vi "PJ1_GG - Sigwork.vi"() -> ()   [LabVIEW 2024]
uses:
  Control 1.ctl
  <vilib>/Instr/_visa.llb/VISA Configure Serial Port (Instr).vi
  <vilib>/express/express analysis/Spectral/Block/exnSpectralBlock spectral measurements PSD poly.vi
  <vilib>/express/express analysis/Spectral/Block/exnSpectralBlock spectral measurements PSD DDT.vi
  <vilib>/express/express analysis/Spectral/XNode/ExpressSpectralMeasurementsBlockNode.xnode
panel:
  out "Array":dbl[](array[numeric])
  out "appended array 2":dbl[](array[numeric])
  out "data out":string
  in  "Sample":i32
  in  "Rate":dbl
  in  "Upper Cut-Off":dbl=40.0
  out "PSD":dynamicdata(graph)
  out "PSD MAX":dbl
  out "Index ที่มากที่สุด":i32
  out "max value":dbl
  out "B 18+1":dbl
  out "N 18+1":dbl
  in  "Aj 18+1":dbl
  out "B 18+1":dbl
  out "PSD 18+1":dbl
  out "B 18":dbl
  out "N 18":dbl
  in  "Aj 18":dbl
  out "B 18":dbl
  out "PSD 18":dbl
  out "B 18-1":dbl
  out "N 18-1":dbl
  in  "Aj 18-1":dbl
  out "B 18-1":dbl
  out "PSD 18-1":dbl
  out "9 Hz":dbl[](array[numeric])
  out "Max Index 9":i32
  out "PSD max 9":dbl
  out "PSD 9-1":dbl
  out "B 9-1":dbl
  in  "Aj 9-1":dbl
  out "N 9-1":dbl
  out "B 9-1":dbl
  out "PSD 9":dbl
  out "B 9":dbl
  in  "Aj 9":dbl
  out "N 9":dbl
  out "B 9":dbl
  out "PSD 9+1":dbl
  out "B 9+1":dbl
  in  "Aj 9+1":dbl
  out "N 9+1":dbl
  out "B 9+1":dbl
  out "8 Hz":dbl[](array[numeric])
  out "Max Index 8":i32
  out "PSD max 8":dbl
  out "B 16+1":dbl
  out "N 16+1":dbl
  in  "Aj  16+1":dbl
  out "B 16+1":dbl
  out "PSD  16+1":dbl
  out "B 16":dbl
  out "N  16":dbl
  in  "Aj  16":dbl
  out "B 16":dbl
  out "PSD  16":dbl
  out "B 16-1":dbl
  out "N  16-1":dbl
  in  "Aj   16-1":dbl
  out "B   16-1":dbl
  out "PSD 16-1":dbl
  out "B 8+1":dbl
  out "N 8+1":dbl
  in  "Aj  8+1":dbl
  out "B  8+1":dbl
  out "PSD 8+1":dbl
  out "B 8":dbl
  out "N  8":dbl
  in  "Aj  8":dbl
  out "B  8":dbl
  out "PSD 8":dbl
  out "B 8-1":dbl
  out "N  8-1":dbl
  in  "Aj  8-1":dbl
  out "B  8-1":dbl
  out "PSD 8-1":dbl
  out "PSD 14+1":dbl
  out "B 14+1":dbl
  in  "Aj 14+1":dbl
  out "N 14+1":dbl
  out "B 14+1":dbl
  out "PSD 14":dbl
  out "B 14":dbl
  in  "Aj 14":dbl
  out "N 14":dbl
  out "B 14":dbl
  out "PSD 14-1":dbl
  out "B 14-1":dbl
  in  "Aj 14-1":dbl
  out "N 14-1":dbl
  out "B 14-1":dbl
  out "PSD7+1":dbl
  out "B7+1":dbl
  in  "Aj7+1":dbl
  out "N7+1":dbl
  out "B7+1":dbl
  out "PSD 7":dbl
  out "B 7":dbl
  in  "Aj 7":dbl
  out "N7":dbl
  out "B7":dbl
  out "7 Hz":dbl[](array[numeric])
  out "Max Index 7":i32
  out "PSD max 7":dbl
  out "PSD 7-1":dbl
  out "B 7-1":dbl
  in  "Aj 7-1":dbl
  out "N7-1":dbl
  out "B7-1":dbl
  out "B12-1":dbl
  out "N12-1":dbl
  in  "Aj 12-1":dbl
  out "B 12-1":dbl
  out "PSD 12-1":dbl
  out "B12":dbl
  out "N12":dbl
  in  "Aj 12":dbl
  out "B12":dbl
  out "PSD 12":dbl
  out "B12+1":dbl
  out "N12+1":dbl
  in  "Aj 12+1":dbl
  out "B 12+1":dbl
  out "PSD 12+1":dbl
  out "B6+1":dbl
  out "N6+1":dbl
  in  "Aj 6+1":dbl
  out "B 6+1":dbl
  out "PSD 6+1":dbl
  out "B6":dbl
  out "N6":dbl
  in  "Aj 6":dbl
  out "B6":dbl
  out "PSD 6":dbl
  out "PSD 6-1":dbl
  out "6 Hz":dbl[](array[numeric])
  out "Max Index 6":i32
  out "PSD max 6":dbl
  out "B 6-1":dbl
  in  "Aj 6-1":dbl
  out "N6-1":dbl
  out "B6-1":dbl
  in  "Baseline":bool
  out "appended array":dbl[][](array[numeric])
  out "Filtered Signal":dynamicdata(graph)
  in  "Lower Cut-Off":dbl=1.0
  out "?":bool
  out "?":bool
  out "?":bool
  out "?":bool
  out "?":bool
  out "?":bool
  out "?":bool
  out "?":bool
  out "?":bool
  out "?":bool
  out "?":bool=TRUE
  out "?":bool=TRUE
  out "?":bool=TRUE
  out "?":bool=TRUE
  out "?":bool=TRUE
  out "?":bool=TRUE
  out "?":bool=TRUE
  out "?":bool=TRUE
  out "?":bool=TRUE
  out "?":bool=TRUE
  out "?":bool
  out "?":bool
  out "?":bool
  out "?":bool
  out "?":bool
  out "?":bool
  out "?":bool
  out "?":bool
  out "?":bool
  out "?":bool
  out "?":bool=TRUE
  out "?":bool=TRUE
  out "?":bool=TRUE
  out "?":bool=TRUE
  out "?":bool=TRUE
  out "?":bool=TRUE
  out "?":bool=TRUE
  out "?":bool=TRUE
  out "?":bool=TRUE
  out "?":bool=TRUE
  out "?":bool
  out "?":bool
  out "?":bool
  out "?":bool
  out "?":bool
  out "?":bool
  out "?":bool
  out "?":bool
  out "?":bool
  out "?":bool
  out "?":bool=TRUE
  out "?":bool=TRUE
  out "?":bool=TRUE
  out "?":bool=TRUE
  out "?":bool=TRUE
  out "?":bool=TRUE
  out "?":bool=TRUE
  out "?":bool=TRUE
  out "?":bool=TRUE
  out "?":bool=TRUE
  out "?":bool
  out "?":bool
  out "?":bool
  out "?":bool
  out "?":bool
  out "?":bool
  out "?":bool
  out "?":bool
  out "?":bool
  out "?":bool
  out "?":bool=TRUE
  out "?":bool=TRUE
  out "?":bool=TRUE
  out "?":bool=TRUE
  out "?":bool=TRUE
  out "?":bool=TRUE
  out "?":bool=TRUE
  out "?":bool=TRUE
  out "?":bool=TRUE
  out "?":bool=TRUE
  out "9 HZ":bool
  out "8 HZ":bool
  out "6 HZ":bool
  out "7 HZ":bool
  in  "Tab Control":enum32{"TAB 1", "TAB 2", "TAB 3", "TAB 4"}(tab)
  out "555":bool
  in  "MENU 4":bool
  in  "MENU 3":bool
  in  "MENU 2":bool
  in  "MENU":bool
  in  "start":bool
  in  "Text3":bool
  in  "Text2":bool
  in  "Backpage 2":T1
  out "String":string
  in  "Text1":bool
  in  "send":bool
  in  "Back":bool
  in  "1 3":bool
  in  "1 2":bool
  in  "1":bool
  out "String 2":string
  in  "SOS CALLING":bool
  in  "Blank Button 14":bool
  in  "LED":bool
  in  "Blank Button 12":bool
  in  "Back 4":bool
  in  "VISA resource name":refnum<visa-resource-name>
  # "Tel."
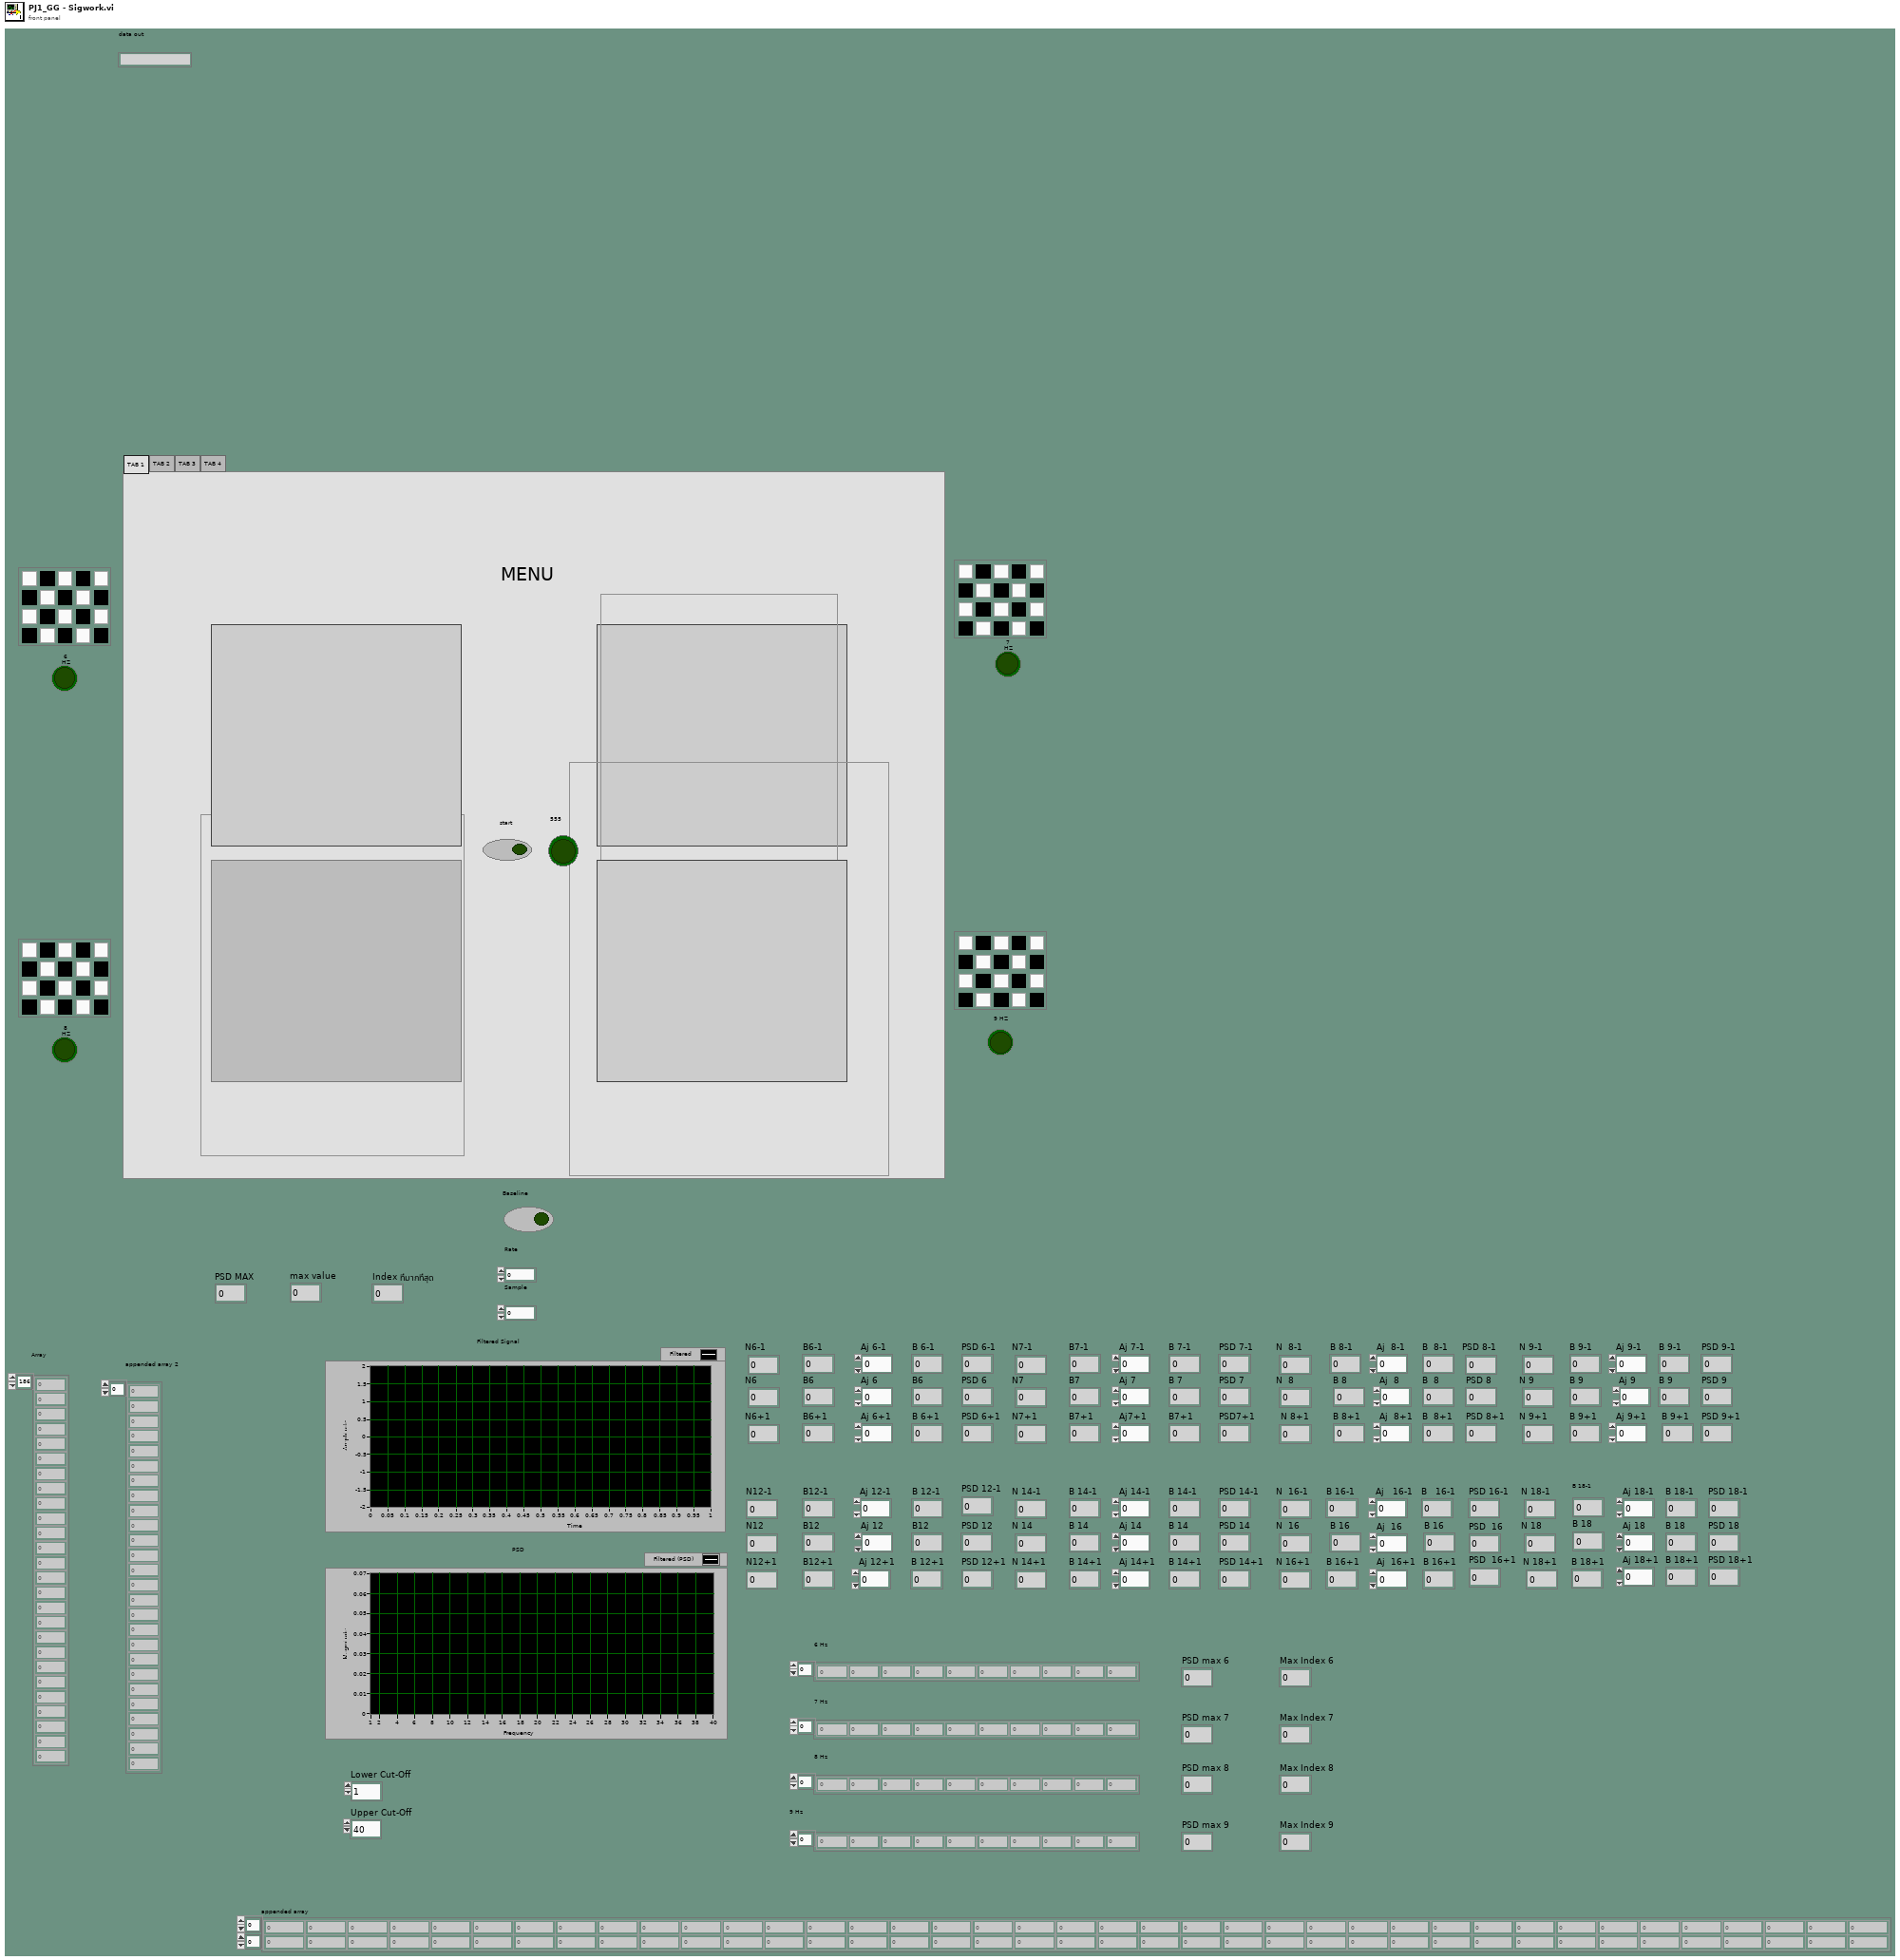
[diagram p1: front panel]
types:
  T1 = typedef "Control 1.ctl" = bool
  T2 = cluster{"averaging mode":u16, "weighting mode":u16, "number of averages":u32}
  T3 = cluster{"dB On (F)":bool, "unwrap phase (F)":bool, "convert to degree (F)":bool}
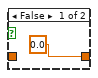
[diagram p3: hidden frame]
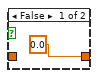
[diagram p5: hidden frame]
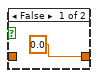
[diagram p7: hidden frame]
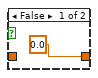
[diagram p9: hidden frame]
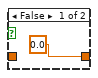
[diagram p11: hidden frame]
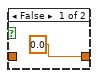
[diagram p13: hidden frame]
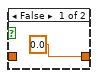
[diagram p15: hidden frame]
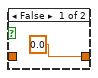
[diagram p17: hidden frame]
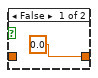
[diagram p19: hidden frame]
diagram:
  n1 = while {
    tunnel: [w15] -> _
    tunnel: [w16] -> _
    stop <- FALSE stop-if-true
    n2 = Obtain Queue(name (unnamed)="buffer", element data type=dbl[] []) -> (queue out=w11:refnum<queue>, error out=w10:errorcluster)  [unwired: 3 in, 1 out]
    n3 = Obtain Queue(name (unnamed)="ganglion", element data type=0.0) -> (queue out=w16:refnum<queue>, error out=w15:errorcluster)  [unwired: 3 in, 1 out]
    n4 = while {
      tunnel: w16 -> [w532]
      tunnel: w15 -> [w531]
      shift-right: [w523] -> _
      shift-left: _ -> [_]
      tunnel: w11 -> [w528]
      tunnel: w10 -> [w527]
      tunnel: [w526] -> w13
      tunnel: [w525] -> w12
      stop <- FALSE stop-if-true
      # "เงื่อนไข while"
      n5 = for {
        N: 200 -> [_]
        shift-right: [w534] -> w523
        shift-left: dbl[] [] -> [w536]
        tunnel: [w541] -> _
        tunnel: w531 -> [w542]
        tunnel: [w538] -> _
        tunnel: [w537] -> _
        tunnel: w532 -> [w541]
        # "เคลีย 800 ก่อน"
        # "ตัด 1 วิเเรกออก"
        n6 = Dequeue Element(queue=w541, error in (no error)=w542) -> (queue out=w537:refnum<queue>, element=w535:dbl, error out=w538:errorcluster)  [unwired: 1 in, 1 out]
        n7 = Build Array (concatenate) "Build Array"(w535, w536) -> (w533:dbl[])
        "appended array 2" <- w533
        n8 = Delete From Array "Delete From Array"(array=w533, length=0, index=199 ("index (row)")) -> (array with subset deleted=w534:dbl[])  [unwired: 1 out]
      }
      "Array" <- w523
      n9 = Enqueue Element(queue=w528, element=w523, error in (no error)=w527) -> (queue out=w526:refnum<queue>, error out=w525:errorcluster)  [unwired: 1 in, 1 out]
    }
    n10 = String To IP(1:"127.0.0.1") -> (0:w21:u32)
    n11 = UDP Open(7:w21, 11:u16 5005 ("port")) -> (port=w23:refnum<k16>, 0:w22:errorcluster)  [unwired: 3 in, 1 out]
    n12 = while {
      tunnel: w22 -> [w560]
      tunnel: w23 -> [w558]
      tunnel: [w557] -> w24
      tunnel: [w556] -> w25
      tunnel: [w550] -> w26
      tunnel: w15 -> [w552]
      tunnel: [w551] -> w27
      tunnel: w16 -> [w553]
      stop <- FALSE stop-if-true
      n13 = UDP Read(connection ID=w558, timeout ms (25000)=500, 8:w560) -> (data out=w549:string, error out=w557:errorcluster, 3:w556:refnum<k16>)  [unwired: 1 in, 2 out]
      "data out" <- w549
      n14 = Spreadsheet String To Array(delimiter (Tab)=",", format string="%f", spreadsheet string=w549, array type (2D Dbl)=0.0) -> (array=w547:dbl[][])
      n15 = Index Array(array=w547, index (row)=0, index (col)=0 ("disabled index (col)")) -> (element=w546:dbl)
      n16 = Enqueue Element(queue=w553, element=w546, error in (no error)=w552) -> (queue out=w550:refnum<queue>, error out=w551:errorcluster)  [unwired: 1 in, 1 out]
    }
    n17 = UDP Close(connection ID=w25, 8:w24) -> ()  [unwired: 2 out]
    n18 = Release Queue(queue=w26, error in (no error)=w27) -> ()  [unwired: 1 in, 3 out]
    n19 = Release Queue(queue=w13, error in (no error)=w12) -> ()  [unwired: 1 in, 3 out]
    n20 = while {
      tunnel: w11 -> [w31]
      tunnel: w10 -> [w30]
      stop <- FALSE stop-if-true
      n21 = Dequeue Element(queue=w31, error in (no error)=w30) -> (element=w29:dbl[])  [unwired: 1 in, 3 out]
      n22 = Bundle By Name("dt"=0.005, "Y"=w29) -> (w33:waveform(dbl))  [unwired: 1 in]
      n23 = Divide(x="Rate", y="Sample") -> (x/y=w126:dbl)
      n24 = call "Filter"("Lower Cut-Off"="Lower Cut-Off", "Upper Cut-Off"="Upper Cut-Off", "Signal"=w33) -> ("Filtered Signal"=w35:dynamicdata)  [unwired: 7 in, 1 out]
      "Filtered Signal" <- w35
      n25 = Divide(x=8.0, y=w126) -> (x/y=w226:dbl)
      n26 = Divide(x=16.0, y=w126) -> (x/y=w178:dbl)
      n27 = Divide(x=14.0, y=w126) -> (x/y=w251:dbl)
      n28 = Divide(x=18.0, y=w126) -> (x/y=w101:dbl)
      n29 = xnode "Spectral Measurements"("Signals"=w35) -> ("PSD"=w36:dynamicdata)  [unwired: 1 in, 1 out]
      "PSD" <- w36
      n30 = Divide(x=9.0, y=w126) -> (x/y=w144:dbl)
      n31 = Divide(x=7.0, y=w126) -> (x/y=w268:dbl)
      n32 = Divide(x=12.0, y=w126) -> (x/y=w337:dbl)
      n33 = Divide(x=6.0, y=w126) -> (x/y=w386:dbl)
      n34 = Decrement(x=w144) -> (x-1=w175:dbl)
      n35 = Increment(x=w144) -> (x+1=w143:dbl)
      n36 = call "Convert from Dynamic Data"("Dynamic Data Type"=w36) -> ("Array"=w414:dbl[])  [unwired: 3 in]
      n37 = Increment(x=w101) -> (x+1=w90:dbl)
      n38 = Decrement(x=w101) -> (x-1=w115:dbl)
      n39 = Decrement(x=w251) -> (x-1=w280:dbl)
      n40 = Increment(x=w226) -> (x+1=w216:dbl)
      n41 = Decrement(x=w178) -> (x-1=w201:dbl)
      n42 = Decrement(x=w386) -> (x-1=w399:dbl)
      n43 = Decrement(x=w268) -> (x-1=w309:dbl)
      "PSD 7-1" <- w309
      n44 = Increment(x=w268) -> (x+1=w294:dbl)
      n45 = Decrement(x=w226) -> (x-1=w239:dbl)
      n46 = Increment(x=w178) -> (x+1=w177:dbl)
      n47 = Increment(x=w386) -> (x+1=w375:dbl)
      n48 = Increment(x=w251) -> (x+1=w257:dbl)
      n49 = Decrement(x=w337) -> (x-1=w342:dbl)
      n50 = Increment(x=w337) -> (x+1=w336:dbl)
      n51 = Build Array "Build Array"(w414) -> (w91:dbl[][])
      "appended array" <- w91
      n52 = Index Array(array=w91, index (row)=0, index (col)=w201) -> (element=w212:dbl)
      "PSD 16-1" <- w212
      n53 = Index Array(array=w91, index (row)=0 ("disabled index (row)"), index (col)=w177) -> (element=w189:dbl)
      "PSD  16+1" <- w189
      n54 = Index Array(array=w91, index (row)=0 ("disabled index (row)"), index (col)=w178) -> (element=w191:dbl)
      "PSD  16" <- w191
      n55 = Index Array(array=w91, index (row)=0, index (col)=w257) -> (element=w258:dbl)
      "PSD 14+1" <- w258
      n56 = Index Array(array=w91, index (row)=0 ("disabled index (row)"), index (col)=w115) -> (element=w113:dbl)
      "PSD 18-1" <- w113
      n57 = Index Array(array=w91, index (row)=0, index (col)=w216) -> (element=w214:dbl)
      "PSD 8+1" <- w214
      n58 = Index Array(array=w91, index (row)=0 ("disabled index (row)"), index (col)=w90) -> (element=w87:dbl)
      "PSD 18+1" <- w87
      n59 = Index Array(array=w91, index (row)=0, index (col)=w143) -> (element=w132:dbl)
      "PSD 9-1" <- w132
      n60 = Index Array(array=w91, index (row)=0, index (col)=w226) -> (element=w237:dbl)
      "PSD 8" <- w237
      n61 = Index Array(array=w91, index (row)=0 ("disabled index (row)"), index (col)=w101) -> (element=w102:dbl)
      "PSD 18" <- w102
      n62 = Index Array(array=w91, index (row)=0, index (col)=w239) -> (element=w238:dbl)
      "PSD 8-1" <- w238
      n63 = Index Array(array=w91, index (row)=0, index (col)=w144) -> (element=w145:dbl)
      "PSD 9" <- w145
      n64 = Index Array(array=w91, index (row)=0, index (col)=w175) -> (element=w156:dbl)
      "PSD 9+1" <- w156
      n65 = Index Array(array=w91, index (row)=0, index (col)=w280) -> (element=w282:dbl)
      "PSD 14-1" <- w282
      n66 = Index Array(array=w91, index (row)=0, index (col)=w251) -> (element=w269:dbl)
      "PSD 14" <- w269
      n67 = Index Array(array=w91, index (row)=0, index (col)=w309) -> ()  [unwired: 1 out]
      n68 = Index Array(array=w91, index (row)=0 ("disabled index (row)"), index (col)=w268) -> (element=w306:dbl)
      "PSD 7" <- w306
      n69 = Index Array(array=w91, index (row)=0, index (col)=w294) -> (element=w295:dbl)
      "PSD7+1" <- w295
      n70 = Index Array(array=w91, index (row)=0 ("disabled index (row)"), index (col)=w375) -> (element=w373:dbl)
      "PSD 6+1" <- w373
      n71 = Index Array(array=w91, index (row)=0, index (col)=w342) -> (element=w341:dbl)
      "PSD 12-1" <- w341
      n72 = Index Array(array=w91, index (row)=0 ("disabled index (row)"), index (col)=w337) -> (element=w338:dbl)
      "PSD 12" <- w338
      n73 = Index Array(array=w91, index (row)=0 ("disabled index (row)"), index (col)=w336) -> (element=w334:dbl)
      "PSD 12+1" <- w334
      n74 = Index Array(array=w91, index (row)=0, index (col)=w386) -> (element=w387:dbl)
      "PSD 6" <- w387
      n75 = Index Array(array=w91, index (row)=0, index (col)=w399) -> (element=w406:dbl)
      "PSD 6-1" <- w406
      n76 = feedback #1() -> (w41:dbl)  [unwired: 1 in]
      "B 18" <- w41
      n77 = case shown="False" "Baseline" {
        tunnel: w102 -> [_ w425]
        tunnel: [w424 w425] -> w104
        tunnel: w41 -> [w424 _]
        frame False {
        }
        frame True {
        }
      }
      n78 = feedback-in #1(w104) -> ()
      n79 = feedback #2() -> (w42:dbl)  [unwired: 1 in]
      "B 18-1" <- w42
      n80 = case shown="False" "Baseline" {
        tunnel: w113 -> [_ w429]
        tunnel: [w428 w429] -> w124
        tunnel: w42 -> [w428 _]
        frame False {
        }
        frame True {
        }
      }
      n81 = feedback-in #2(w124) -> ()
      n82 = feedback #3() -> (w40:dbl)  [unwired: 1 in]
      "B 18+1" <- w40
      n83 = case shown="False" "Baseline" {
        tunnel: w87 -> [_ w421]
        tunnel: [w420 w421] -> w100
        tunnel: w40 -> [w420 _]
        frame False {
        }
        frame True {
        }
      }
      n84 = feedback-in #3(w100) -> ()
      n85 = feedback #4() -> (w48:dbl)  [unwired: 1 in]
      "B 16-1" <- w48
      n86 = case shown="True" "Baseline" {
        tunnel: w212 -> [_ w453]
        tunnel: [w452 w453] -> w202
        tunnel: w48 -> [w452 _]
        frame False {
        }
        frame True {
        }
      }
      n87 = feedback-in #4(w202) -> ()
      n88 = feedback #5() -> (w46:dbl)  [unwired: 1 in]
      "B 16+1" <- w46
      n89 = case shown="False" "Baseline" {
        tunnel: w189 -> [_ w445]
        tunnel: [w444 w445] -> w180
        tunnel: w46 -> [w444 _]
        frame False {
        }
        frame True {
        }
      }
      n90 = feedback-in #5(w180) -> ()
      n91 = feedback #6() -> (w47:dbl)  [unwired: 1 in]
      "B 16" <- w47
      n92 = case shown="False" "Baseline" {
        tunnel: w191 -> [_ w449]
        tunnel: [w448 w449] -> w200
        tunnel: w47 -> [w448 _]
        frame False {
        }
        frame True {
        }
      }
      n93 = feedback-in #6(w200) -> ()
      n94 = feedback #7() -> (w49:dbl)  [unwired: 1 in]
      "B 8+1" <- w49
      n95 = case shown="True" "Baseline" {
        tunnel: w214 -> [_ w457]
        tunnel: [w456 w457] -> w225
        tunnel: w49 -> [w456 _]
        frame False {
        }
        frame True {
        }
      }
      n96 = feedback-in #7(w225) -> ()
      n97 = feedback #8() -> (w52:dbl)  [unwired: 1 in]
      "B 14+1" <- w52
      n98 = case shown="True" "Baseline" {
        tunnel: w258 -> [_ w469]
        tunnel: [w468 w469] -> w259
        tunnel: w52 -> [w468 _]
        frame False {
        }
        frame True {
        }
      }
      n99 = feedback-in #8(w259) -> ()
      n100 = feedback #9() -> (w50:dbl)  [unwired: 1 in]
      "B 8" <- w50
      n101 = case shown="True" "Baseline" {
        tunnel: w237 -> [_ w461]
        tunnel: [w460 w461] -> w228
        tunnel: w50 -> [w460 _]
        frame False {
        }
        frame True {
        }
      }
      n102 = feedback-in #9(w228) -> ()
      n103 = feedback #10() -> (w44:dbl)  [unwired: 1 in]
      "B 9" <- w44
      n104 = case shown="False" "Baseline" {
        tunnel: w145 -> [_ w437]
        tunnel: [w436 w437] -> w146
        tunnel: w44 -> [w436 _]
        frame False {
        }
        frame True {
        }
      }
      n105 = feedback-in #10(w146) -> ()
      n106 = feedback #11() -> (w51:dbl)  [unwired: 1 in]
      "B 8-1" <- w51
      n107 = case shown="True" "Baseline" {
        tunnel: w238 -> [_ w465]
        tunnel: [w464 w465] -> w249
        tunnel: w51 -> [w464 _]
        frame False {
        }
        frame True {
        }
      }
      n108 = feedback-in #11(w249) -> ()
      n109 = feedback #12() -> (w45:dbl)  [unwired: 1 in]
      "B 9+1" <- w45
      n110 = case shown="False" "Baseline" {
        tunnel: w156 -> [_ w441]
        tunnel: [w440 w441] -> w157
        tunnel: w45 -> [w440 _]
        frame False {
        }
        frame True {
        }
      }
      n111 = feedback-in #12(w157) -> ()
      n112 = feedback #13() -> (w60:dbl)  [unwired: 1 in]
      "B12-1" <- w60
      n113 = case shown="True" "Baseline" {
        tunnel: w341 -> [_ w501]
        tunnel: [w500 w501] -> w353
        tunnel: w60 -> [w500 _]
        frame False {
        }
        frame True {
        }
      }
      n114 = feedback-in #13(w353) -> ()
      n115 = feedback #14() -> (w54:dbl)  [unwired: 1 in]
      "B 14-1" <- w54
      n116 = case shown="True" "Baseline" {
        tunnel: w282 -> [_ w477]
        tunnel: [w476 w477] -> w283
        tunnel: w54 -> [w476 _]
        frame False {
        }
        frame True {
        }
      }
      n117 = feedback-in #14(w283) -> ()
      n118 = feedback #15() -> (w43:dbl)  [unwired: 1 in]
      "B 9-1" <- w43
      n119 = case shown="False" "Baseline" {
        tunnel: w132 -> [_ w433]
        tunnel: [w432 w433] -> w133
        tunnel: w43 -> [w432 _]
        frame False {
        }
        frame True {
        }
      }
      n120 = feedback-in #15(w133) -> ()
      n121 = feedback #16() -> (w61:dbl)  [unwired: 1 in]
      "B6+1" <- w61
      n122 = case shown="True" "Baseline" {
        tunnel: w373 -> [_ w505]
        tunnel: [w504 w505] -> w376
        tunnel: w61 -> [w504 _]
        frame False {
        }
        frame True {
        }
      }
      n123 = feedback-in #16(w376) -> ()
      n124 = feedback #17() -> (w62:dbl)  [unwired: 1 in]
      "B6" <- w62
      n125 = case shown="True" "Baseline" {
        tunnel: w387 -> [_ w509]
        tunnel: [w508 w509] -> w397
        tunnel: w62 -> [w508 _]
        frame False {
        }
        frame True {
        }
      }
      n126 = feedback-in #17(w397) -> ()
      n127 = feedback #18() -> (w63:dbl)  [unwired: 1 in]
      "B6-1" <- w63
      n128 = case shown="True" "Baseline" {
        tunnel: w406 -> [_ w513]
        tunnel: [w512 w513] -> w398
        tunnel: w63 -> [w512 _]
        frame False {
        }
        frame True {
        }
      }
      n129 = feedback-in #18(w398) -> ()
      n130 = feedback #19() -> (w53:dbl)  [unwired: 1 in]
      "B 14" <- w53
      n131 = case shown="True" "Baseline" {
        tunnel: w269 -> [_ w473]
        tunnel: [w472 w473] -> w271
        tunnel: w53 -> [w472 _]
        frame False {
        }
        frame True {
        }
      }
      n132 = feedback-in #19(w271) -> ()
      n133 = feedback #20() -> (w58:dbl)  [unwired: 1 in]
      "B12+1" <- w58
      n134 = case shown="True" "Baseline" {
        tunnel: w334 -> [_ w493]
        tunnel: [w492 w493] -> w371
        tunnel: w58 -> [w492 _]
        frame False {
        }
        frame True {
        }
      }
      n135 = feedback-in #20(w371) -> ()
      n136 = Add(x=w41, y="Aj 18") -> (x+y=w108:dbl)
      "B 18" <- w108
      n137 = Add(x=w42, y="Aj 18-1") -> (x+y=w120:dbl)
      "B 18-1" <- w120
      n138 = Add(x=w40, y="Aj 18+1") -> (x+y=w96:dbl)
      "B 18+1" <- w96
      n139 = feedback #21() -> (w59:dbl)  [unwired: 1 in]
      "B12" <- w59
      n140 = case shown="True" "Baseline" {
        tunnel: w338 -> [_ w497]
        tunnel: [w496 w497] -> w354
        tunnel: w59 -> [w496 _]
        frame False {
        }
        frame True {
        }
      }
      n141 = feedback-in #21(w354) -> ()
      n142 = Add(x=w48, y="Aj   16-1") -> (x+y=w206:dbl)
      "B   16-1" <- w206
      n143 = Add(x=w46, y="Aj  16+1") -> (x+y=w184:dbl)
      "B 16+1" <- w184
      n144 = Add(x=w47, y="Aj  16") -> (x+y=w196:dbl)
      "B 16" <- w196
      n145 = Add(x=w49, y="Aj  8+1") -> (x+y=w221:dbl)
      "B  8+1" <- w221
      n146 = Add(x=w52, y="Aj 14+1") -> (x+y=w263:dbl)
      "B 14+1" <- w263
      n147 = Add(x=w50, y="Aj  8") -> (x+y=w232:dbl)
      "B  8" <- w232
      n148 = Add(x=w44, y="Aj 9") -> (x+y=w150:dbl)
      "B 9" <- w150
      n149 = Add(x=w51, y="Aj  8-1") -> (x+y=w245:dbl)
      "B  8-1" <- w245
      n150 = Add(x=w45, y="Aj 9+1") -> (x+y=w161:dbl)
      "B 9+1" <- w161
      n151 = Add(x=w60, y="Aj 12-1") -> (x+y=w349:dbl)
      "B 12-1" <- w349
      n152 = Add(x=w54, y="Aj 14-1") -> (x+y=w287:dbl)
      "B 14-1" <- w287
      n153 = Add(x=w43, y="Aj 9-1") -> (x+y=w137:dbl)
      "B 9-1" <- w137
      n154 = Multiply(x=w41, y=5.0) -> (x*y=w111:dbl)
      "N 18" <- w111
      n155 = Add(x=w61, y="Aj 6+1") -> (x+y=w380:dbl)
      "B 6+1" <- w380
      n156 = Multiply(x=w42, y=5.0) -> (x*y=w117:dbl)
      "N 18-1" <- w117
      n157 = Multiply(x=w40, y=5.0) -> (x*y=w93:dbl)
      "N 18+1" <- w93
      n158 = feedback #22() -> (w55:dbl)  [unwired: 1 in]
      "B7+1" <- w55
      n159 = case shown="True" "Baseline" {
        tunnel: w295 -> [_ w481]
        tunnel: [w480 w481] -> w297
        tunnel: w55 -> [w480 _]
        frame False {
        }
        frame True {
        }
      }
      n160 = feedback-in #22(w297) -> ()
      n161 = feedback #23() -> (w56:dbl)  [unwired: 1 in]
      "B7" <- w56
      n162 = case shown="True" "Baseline" {
        tunnel: w306 -> [_ w485]
        tunnel: [w484 w485] -> w310
        tunnel: w56 -> [w484 _]
        frame False {
        }
        frame True {
        }
      }
      n163 = feedback-in #23(w310) -> ()
      n164 = Multiply(x=w48, y=5.0) -> (x*y=w209:dbl)
      "N  16-1" <- w209
      n165 = Multiply(x=w46, y=5.0) -> (x*y=w187:dbl)
      "N 16+1" <- w187
      n166 = Multiply(x=w47, y=5.0) -> (x*y=w193:dbl)
      "N  16" <- w193
      n167 = Multiply(x=w49, y=5.0) -> (x*y=w218:dbl)
      "N 8+1" <- w218
      n168 = feedback #24() -> (w57:dbl)  [unwired: 1 in]
      "B7-1" <- w57
      n169 = case shown="False" "Baseline" {
        tunnel: w309 -> [_ w489]
        tunnel: [w488 w489] -> w323
        tunnel: w57 -> [w488 _]
        frame False {
        }
        frame True {
        }
      }
      n170 = feedback-in #24(w323) -> ()
      n171 = Add(x=w62, y="Aj 6") -> (x+y=w393:dbl)
      "B6" <- w393
      n172 = Add(x=w63, y="Aj 6-1") -> (x+y=w407:dbl)
      "B 6-1" <- w407
      n173 = Add(x=w53, y="Aj 14") -> (x+y=w275:dbl)
      "B 14" <- w275
      n174 = Multiply(x=w52, y=5.0) -> (x*y=w266:dbl)
      "N 14+1" <- w266
      n175 = Multiply(x=w50, y=5.0) -> (x*y=w235:dbl)
      "N  8" <- w235
      n176 = Multiply(x=w44, y=5.0) -> (x*y=w153:dbl)
      "N 9" <- w153
      n177 = Multiply(x=w51, y=5.0) -> (x*y=w242:dbl)
      "N  8-1" <- w242
      n178 = Multiply(x=w45, y=5.0) -> (x*y=w164:dbl)
      "N 9+1" <- w164
      n179 = Add(x=w58, y="Aj 12+1") -> (x+y=w367:dbl)
      "B 12+1" <- w367
      n180 = Multiply(x=w60, y=5.0) -> (x*y=w346:dbl)
      "N12-1" <- w346
      n181 = Multiply(x=w54, y=5.0) -> (x*y=w290:dbl)
      "N 14-1" <- w290
      n182 = Add(x=w59, y="Aj 12") -> (x+y=w358:dbl)
      "B12" <- w358
      n183 = Multiply(x=w43, y=5.0) -> (x*y=w140:dbl)
      "N 9-1" <- w140
      n184 = Multiply(x=w61, y=5.0) -> (x*y=w383:dbl)
      "N6+1" <- w383
      n185 = Greater?(x=w102, y=w108) -> (0:w109:bool)
      n186 = Greater?(x=w113, y=w120) -> (0:w119:bool)
      n187 = Greater?(x=w87, y=w96) -> (0:w95:bool)
      n188 = Less?(x=w102, y=w111) -> (x < y?=w110:bool)
      n189 = Less?(x=w113, y=w117) -> (x < y?=w118:bool)
      n190 = Multiply(x=w62, y=5.0) -> (x*y=w390:dbl)
      "N6" <- w390
      n191 = Multiply(x=w63, y=5.0) -> (x*y=w410:dbl)
      "N6-1" <- w410
      n192 = Multiply(x=w53, y=5.0) -> (x*y=w278:dbl)
      "N 14" <- w278
      n193 = Greater?(x=w212, y=w206) -> (0:w207:bool)
      n194 = Less?(x=w87, y=w93) -> (x < y?=w94:bool)
      n195 = Greater?(x=w189, y=w184) -> (0:w185:bool)
      n196 = Greater?(x=w191, y=w196) -> (0:w195:bool)
      n197 = Greater?(x=w214, y=w221) -> (0:w220:bool)
      n198 = Less?(x=w212, y=w209) -> (x < y?=w208:bool)
      n199 = Less?(x=w189, y=w187) -> (x < y?=w186:bool)
      n200 = Multiply(x=w58, y=5.0) -> (x*y=w364:dbl)
      "N12+1" <- w364
      n201 = Less?(x=w191, y=w193) -> (x < y?=w194:bool)
      n202 = Greater?(x=w258, y=w263) -> (0:w264:bool)
      n203 = Less?(x=w214, y=w218) -> (x < y?=w219:bool)
      n204 = Greater?(x=w237, y=w232) -> (0:w233:bool)
      n205 = Greater?(x=w145, y=w150) -> (0:w151:bool)
      n206 = Multiply(x=w59, y=5.0) -> (x*y=w361:dbl)
      "N12" <- w361
      n207 = Add(x=w55, y="Aj7+1") -> (x+y=w301:dbl)
      "B7+1" <- w301
      n208 = Less?(x=w258, y=w266) -> (x < y?=w265:bool)
      n209 = Greater?(x=w238, y=w245) -> (0:w244:bool)
      n210 = Less?(x=w237, y=w235) -> (x < y?=w234:bool)
      n211 = Less?(x=w145, y=w153) -> (x < y?=w152:bool)
      n212 = Greater?(x=w156, y=w161) -> (0:w162:bool)
      n213 = Add(x=w56, y="Aj 7") -> (x+y=w314:dbl)
      "B 7" <- w314
      n214 = Less?(x=w238, y=w242) -> (x < y?=w243:bool)
      n215 = Greater?(x=w341, y=w349) -> (0:w348:bool)
      n216 = Greater?(x=w282, y=w287) -> (0:w288:bool)
      n217 = Less?(x=w156, y=w164) -> (x < y?=w163:bool)
      n218 = Greater?(x=w132, y=w137) -> (0:w138:bool)
      n219 = Add(x=w57, y="Aj 7-1") -> (x+y=w327:dbl)
      "B 7-1" <- w327
      n220 = Greater?(x=w373, y=w380) -> (0:w381:bool)
      n221 = Less?(x=w341, y=w346) -> (x < y?=w347:bool)
      n222 = Less?(x=w282, y=w290) -> (x < y?=w289:bool)
      n223 = Less?(x=w132, y=w140) -> (x < y?=w139:bool)
      n224 = Less?(x=w373, y=w383) -> (x < y?=w382:bool)
      n225 = And(x=w110, y=w109) -> (x .and. y?=w107:bool)
      n226 = Subtract(x=w102, y=w108) -> (x-y=w106:dbl)
      n227 = And(x=w118, y=w119) -> (x .and. y?=w121:bool)
      n228 = Greater?(x=w387, y=w393) -> (0:w392:bool)
      n229 = Subtract(x=w113, y=w120) -> (x-y=w122:dbl)
      n230 = Greater?(x=w406, y=w407) -> (0:w408:bool)
      n231 = Greater?(x=w269, y=w275) -> (0:w276:bool)
      n232 = And(x=w94, y=w95) -> (x .and. y?=w97:bool)
      n233 = Subtract(x=w87, y=w96) -> (x-y=w98:dbl)
      n234 = Less?(x=w387, y=w390) -> (x < y?=w391:bool)
      n235 = Less?(x=w406, y=w410) -> (x < y?=w409:bool)
      n236 = Less?(x=w269, y=w278) -> (x < y?=w277:bool)
      n237 = And(x=w208, y=w207) -> (x .and. y?=w205:bool)
      n238 = Multiply(x=w55, y=5.0) -> (x*y=w304:dbl)
      "N7+1" <- w304
      n239 = Subtract(x=w212, y=w206) -> (x-y=w204:dbl)
      n240 = And(x=w186, y=w185) -> (x .and. y?=w183:bool)
      n241 = Subtract(x=w189, y=w184) -> (x-y=w182:dbl)
      n242 = Greater?(x=w334, y=w367) -> (0:w366:bool)
      n243 = Multiply(x=w56, y=5.0) -> (x*y=w317:dbl)
      "N7" <- w317
      n244 = And(x=w194, y=w195) -> (x .and. y?=w197:bool)
      n245 = And(x=w219, y=w220) -> (x .and. y?=w222:bool)
      n246 = Subtract(x=w191, y=w196) -> (x-y=w198:dbl)
      n247 = Subtract(x=w214, y=w221) -> (x-y=w223:dbl)
      n248 = Greater?(x=w338, y=w358) -> (0:w359:bool)
      n249 = Less?(x=w334, y=w364) -> (x < y?=w365:bool)
      n250 = And(x=w265, y=w264) -> (x .and. y?=w262:bool)
      n251 = Subtract(x=w258, y=w263) -> (x-y=w261:dbl)
      n252 = Multiply(x=w57, y=5.0) -> (x*y=w330:dbl)
      "N7-1" <- w330
      n253 = And(x=w234, y=w233) -> (x .and. y?=w231:bool)
      n254 = Subtract(x=w237, y=w232) -> (x-y=w230:dbl)
      n255 = And(x=w152, y=w151) -> (x .and. y?=w149:bool)
      n256 = Subtract(x=w145, y=w150) -> (x-y=w148:dbl)
      n257 = Less?(x=w338, y=w361) -> (x < y?=w360:bool)
      n258 = And(x=w243, y=w244) -> (x .and. y?=w246:bool)
      n259 = Subtract(x=w238, y=w245) -> (x-y=w247:dbl)
      n260 = And(x=w163, y=w162) -> (x .and. y?=w160:bool)
      n261 = Subtract(x=w156, y=w161) -> (x-y=w159:dbl)
      n262 = And(x=w347, y=w348) -> (x .and. y?=w350:bool)
      n263 = Subtract(x=w341, y=w349) -> (x-y=w351:dbl)
      n264 = And(x=w289, y=w288) -> (x .and. y?=w286:bool)
      n265 = Subtract(x=w282, y=w287) -> (x-y=w285:dbl)
      n266 = And(x=w139, y=w138) -> (x .and. y?=w136:bool)
      n267 = Subtract(x=w132, y=w137) -> (x-y=w135:dbl)
      n268 = Subtract(x=w373, y=w380) -> (x-y=w378:dbl)
      n269 = And(x=w382, y=w381) -> (x .and. y?=w379:bool)
      n270 = And(x=w409, y=w408) -> (x .and. y?=w405:bool)
      n271 = Subtract(x=w387, y=w393) -> (x-y=w395:dbl)
      n272 = And(x=w277, y=w276) -> (x .and. y?=w274:bool)
      n273 = Subtract(x=w406, y=w407) -> (x-y=w404:dbl)
      n274 = Greater?(x=w295, y=w301) -> (0:w302:bool)
      n275 = Subtract(x=w269, y=w275) -> (x-y=w273:dbl)
      n276 = Greater?(x=w306, y=w314) -> (0:w315:bool)
      n277 = And(x=w391, y=w392) -> (x .and. y?=w394:bool)
      n278 = Less?(x=w295, y=w304) -> (x < y?=w303:bool)
      n279 = Less?(x=w306, y=w317) -> (x < y?=w316:bool)
      n280 = Subtract(x=w334, y=w367) -> (x-y=w369:dbl)
      n281 = Greater?(x=w309, y=w327) -> (0:w328:bool)
      n282 = Subtract(x=w338, y=w358) -> (x-y=w356:dbl)
      n283 = And(x=w365, y=w366) -> (x .and. y?=w368:bool)
      n284 = Less?(x=w309, y=w330) -> (x < y?=w329:bool)
      n285 = And(x=w360, y=w359) -> (x .and. y?=w357:bool)
      n286 = And(x=w303, y=w302) -> (x .and. y?=w300:bool)
      n287 = Subtract(x=w295, y=w301) -> (x-y=w299:dbl)
      n288 = And(x=w316, y=w315) -> (x .and. y?=w313:bool)
      n289 = Subtract(x=w306, y=w314) -> (x-y=w312:dbl)
      n290 = And(x=w329, y=w328) -> (x .and. y?=w326:bool)
      n291 = Subtract(x=w309, y=w327) -> (x-y=w325:dbl)
      n292 = case shown="True" w350 {
        tunnel: w351 -> [_ w499]
        tunnel: [0.0 w499] -> w340
        frame False {
        }
        frame True {
        }
      }
      n293 = case shown="True" w379 {
        tunnel: w378 -> [_ w503]
        tunnel: [0.0 w503] -> w372
        frame False {
        }
        frame True {
        }
      }
      n294 = case shown="True" w405 {
        tunnel: w404 -> [_ w511]
        tunnel: [0.0 w511] -> w402
        frame False {
        }
        frame True {
        }
      }
      n295 = case shown="False" w394 {
        tunnel: w395 -> [_ w507]
        tunnel: [0.0 w507] -> w385
        frame False {
        }
        frame True {
        }
      }
      n296 = case shown="True" w368 {
        tunnel: w369 -> [_ w491]
        tunnel: [0.0 w491] -> w332
        frame False {
        }
        frame True {
        }
      }
      n297 = case shown="True" w107 {
        tunnel: w106 -> [_ w423]
        tunnel: [0.0 w423] -> w85
        frame False {
        }
        frame True {
        }
      }
      n298 = case shown="True" w357 {
        tunnel: w356 -> [_ w495]
        tunnel: [0.0 w495] -> w333
        frame False {
        }
        frame True {
        }
      }
      n299 = case shown="True" w121 {
        tunnel: w122 -> [_ w427]
        tunnel: [0.0 w427] -> w86
        frame False {
        }
        frame True {
        }
      }
      n300 = case shown="True" w97 {
        tunnel: w98 -> [_ w419]
        tunnel: [0.0 w419] -> w84
        frame False {
        }
        frame True {
        }
      }
      n301 = case shown="True" w205 {
        tunnel: w204 -> [_ w451]
        tunnel: [0.0 w451] -> w168
        frame False {
        }
        frame True {
        }
      }
      n302 = case shown="True" w183 {
        tunnel: w182 -> [_ w443]
        tunnel: [0.0 w443] -> w166
        frame False {
        }
        frame True {
        }
      }
      n303 = case shown="True" w197 {
        tunnel: w198 -> [_ w447]
        tunnel: [0.0 w447] -> w167
        frame False {
        }
        frame True {
        }
      }
      n304 = case shown="True" w222 {
        tunnel: w223 -> [_ w455]
        tunnel: [0.0 w455] -> w169
        frame False {
        }
        frame True {
        }
      }
      n305 = case shown="True" w262 {
        tunnel: w261 -> [_ w467]
        tunnel: [0.0 w467] -> w253
        frame False {
        }
        frame True {
        }
      }
      n306 = case shown="True" w231 {
        tunnel: w230 -> [_ w459]
        tunnel: [0.0 w459] -> w170
        frame False {
        }
        frame True {
        }
      }
      n307 = case shown="True" w274 {
        tunnel: w273 -> [_ w471]
        tunnel: [0.0 w471] -> w254
        frame False {
        }
        frame True {
        }
      }
      n308 = case shown="True" w149 {
        tunnel: w148 -> [_ w435]
        tunnel: [0.0 w435] -> w128
        frame False {
        }
        frame True {
        }
      }
      n309 = case shown="True" w246 {
        tunnel: w247 -> [_ w463]
        tunnel: [0.0 w463] -> w171
        frame False {
        }
        frame True {
        }
      }
      n310 = case shown="True" w286 {
        tunnel: w285 -> [_ w475]
        tunnel: [0.0 w475] -> w255
        frame False {
        }
        frame True {
        }
      }
      n311 = case shown="True" w300 {
        tunnel: w299 -> [_ w479]
        tunnel: [0.0 w479] -> w292
        frame False {
        }
        frame True {
        }
      }
      n312 = case shown="True" w160 {
        tunnel: w159 -> [_ w439]
        tunnel: [0.0 w439] -> w129
        frame False {
        }
        frame True {
        }
      }
      n313 = case shown="True" w313 {
        tunnel: w312 -> [_ w483]
        tunnel: [0.0 w483] -> w293
        frame False {
        }
        frame True {
        }
      }
      n314 = case shown="True" w136 {
        tunnel: w135 -> [_ w431]
        tunnel: [0.0 w431] -> w127
        frame False {
        }
        frame True {
        }
      }
      n315 = case shown="False" w326 {
        tunnel: w325 -> [_ w487]
        tunnel: [0.0 w487] -> w319
        frame False {
        }
        frame True {
        }
      }
      n316 = Build Array(w319, w293, w292, w255, w254, w253) -> (w320:dbl[])
      "7 Hz" <- w320
      n317 = Build Array(w402, w385, w372, w340, w333, w332) -> (w400:dbl[])
      "6 Hz" <- w400
      n318 = Array Max & Min(array=w320) -> (max value=w83:dbl, max index (indices)=→"Max Index 7":i32)  [unwired: 2 out]
      "PSD max 7" <- w83
      n319 = Array Max & Min(array=w400) -> (max value=w80:dbl, max index (indices)=→"Max Index 6":i32)  [unwired: 2 out]
      "PSD max 6" <- w80
      n320 = Build Array(w171, w170, w169, w168, w167, w166) -> (w172:dbl[])
      "8 Hz" <- w172
      n321 = Build Array(w129, w128, w127, w86, w85, w84) -> (w130:dbl[])
      "9 Hz" <- w130
      n322 = Array Max & Min(array=w172) -> (max value=w82:dbl, max index (indices)=→"Max Index 8":i32)  [unwired: 2 out]
      "PSD max 8" <- w82
      n323 = Array Max & Min(array=w130) -> (max value=w81:dbl, max index (indices)=→"Max Index 9":i32)  [unwired: 2 out]
      "PSD max 9" <- w81
      n324 = Build Array(w80, w83, w82, w81) -> (w79:dbl[])
      n325 = Array Max & Min(array=w79) -> (max value=w77:dbl, max index (indices)=w78:i32)  [unwired: 2 out]
      "max value" <- w77
      "PSD MAX" <- w77
      n326 = Greater?(x=w77, y=0.0 ("x")) -> (0:w75:bool)
      n327 = case shown="False" w75 {
        tunnel: w78 -> [_ w417]
        tunnel: [555 w417] -> w65
        frame False {
        }
        frame True {
        }
      }
      "Index ที่มากที่สุด" <- w65
      n328 = Equal?(x=0, y=w65) -> (x = y?=→"6 HZ":bool)
      n329 = Equal?(x=1, y=w65) -> (x = y?=→"7 HZ":bool)
      n330 = Equal?(x=2, y=w65) -> (x = y?=→"9 HZ":bool)
      n331 = Equal?(x=3, y=w65) -> (x = y?=→"8 HZ":bool)
      n332 = Equal?(x=555, y=w65) -> (x = y?=→"555":bool)
    }
  }
  n333 = while {
    shift-right: [w561] -> _
    shift-left: "" -> [w563]
    stop <- FALSE stop-if-true
    n334 = event shown="[3] \"Back\": Value Change" {
      selector: _ -> [_ _ _ _]
      dyn-events: _ -> [_ _ _ _]
      timeout: _ -> [_ _ _ _]
      tunnel: w563 -> [_ _ _ _]
      tunnel: ["0622436287" "1669" " 0937529340" _] -> w561
      event "1 2": Value Change {
        n335 = event-data() -> ()  [unwired: 1 in, 6 out]
      }
      event "1": Value Change {
        n336 = event-data() -> ()  [unwired: 1 in, 6 out]
      }
      event "1 3": Value Change {
        n337 = event-data() -> ()  [unwired: 1 in, 6 out]
      }
      event "Back": Value Change {
        n338 = event-data() -> ()  [unwired: 1 in, 6 out]
        n339 = local write "Tab Control"(enum32{"TAB 1", "TAB 2", "TAB 3", "TAB 4"}."TAB 1" ("Tab Control")) -> ()
      }
    }
    "String 2" <- w561
  }
  n340 = while {
    stop <- FALSE stop-if-true
    n341 = while {
      tunnel: "start" -> [_]
      stop <- FALSE stop-if-true
      n342 = while {
        stop <- FALSE stop-if-true
        w608 = 83.3333
        # "6 HZ"
        n343 = for {
          N: 2 -> [_]
          tunnel: w608 -> [w612]
          i -> [w614]
          n344 = Wait (ms)(milliseconds to wait=w612) -> ()  [unwired: 1 out]
          n345 = Equal?(x=0, y=w614) -> (x = y?=→"?" →"?" →"?" →"?" →"?" →"?" →"?" →"?" →"?" →"?":bool)
        }
        n346 = for {
          N: 2 -> [_]
          tunnel: w608 -> [w616]
          i -> [w617]
          n347 = Wait (ms)(milliseconds to wait=w616) -> ()  [unwired: 1 out]
          n348 = Equal?(x=1, y=w617) -> (x = y?=→"?" →"?" →"?" →"?" →"?" →"?" →"?" →"?" →"?" →"?":bool)
        }
      }
      n349 = while {
        stop <- FALSE stop-if-true
        w596 = 71.428571
        # "7 HZ"
        n350 = for {
          N: 2 -> [_]
          tunnel: w596 -> [w600]
          i -> [w602]
          n351 = Wait (ms)(milliseconds to wait=w600) -> ()  [unwired: 1 out]
          n352 = Equal?(x=0, y=w602) -> (x = y?=→"?" →"?" →"?" →"?" →"?" →"?" →"?" →"?" →"?" →"?":bool)
        }
        n353 = for {
          N: 2 -> [_]
          tunnel: w596 -> [w604]
          i -> [w605]
          n354 = Wait (ms)(milliseconds to wait=w604) -> ()  [unwired: 1 out]
          n355 = Equal?(x=1, y=w605) -> (x = y?=→"?" →"?" →"?" →"?" →"?" →"?" →"?" →"?" →"?" →"?":bool)
        }
      }
      n356 = while {
        stop <- FALSE stop-if-true
        w584 = 62.5
        # "8 HZ"
        n357 = for {
          N: 2 -> [_]
          tunnel: w584 -> [w588]
          i -> [w590]
          n358 = Wait (ms)(milliseconds to wait=w588) -> ()  [unwired: 1 out]
          n359 = Equal?(x=0, y=w590) -> (x = y?=→"?" →"?" →"?" →"?" →"?" →"?" →"?" →"?" →"?" →"?":bool)
        }
        n360 = for {
          N: 2 -> [_]
          tunnel: w584 -> [w592]
          i -> [w593]
          n361 = Wait (ms)(milliseconds to wait=w592) -> ()  [unwired: 1 out]
          n362 = Equal?(x=1, y=w593) -> (x = y?=→"?" →"?" →"?" →"?" →"?" →"?" →"?" →"?" →"?" →"?":bool)
        }
      }
      n363 = while {
        stop <- FALSE stop-if-true
        w572 = 55.5555
        # "9 HZ"
        n364 = for {
          N: 2 -> [_]
          tunnel: w572 -> [w576]
          i -> [w578]
          n365 = Wait (ms)(milliseconds to wait=w576) -> ()  [unwired: 1 out]
          n366 = Equal?(x=0, y=w578) -> (x = y?=→"?" →"?" →"?" →"?" →"?" →"?" →"?" →"?" →"?" →"?":bool)
        }
        n367 = for {
          N: 2 -> [_]
          tunnel: w572 -> [w580]
          i -> [w581]
          n368 = Wait (ms)(milliseconds to wait=w580) -> ()  [unwired: 1 out]
          n369 = Equal?(x=1, y=w581) -> (x = y?=→"?" →"?" →"?" →"?" →"?" →"?" →"?" →"?" →"?" →"?":bool)
        }
      }
    }
  }
  n370 = while {
    stop <- FALSE stop-if-true
    n371 = event shown="[3] \"MENU 2\": Value Change" {
      selector: _ -> [_ _ _ _ _ _ _]
      dyn-events: _ -> [_ _ _ _ _ _ _]
      timeout: _ -> [_ _ _ _ _ _ _]
      event Timeout {
        n372 = event-data() -> ()  [unwired: 1 in, 3 out]
      }
      event "MENU": Value Change {
        n373 = event-data() -> ()  [unwired: 1 in, 6 out]
        n374 = local write "Tab Control"(enum32{"TAB 1", "TAB 2", "TAB 3", "TAB 4"}."TAB 2" ("Tab Control")) -> ()
      }
      event Value Change {
        n375 = event-data() -> ()  [unwired: 1 in, 6 out]
        n376 = local write "Tab Control"(enum32{"TAB 1", "TAB 2", "TAB 3", "TAB 4"}."TAB 1" ("Tab Control")) -> ()
      }
      event "MENU 2": Value Change {
        n377 = event-data() -> ()  [unwired: 1 in, 6 out]
        n378 = local write "Tab Control"(enum32{"TAB 1", "TAB 2", "TAB 3", "TAB 4"}."TAB 3" ("Tab Control")) -> ()
      }
      event "MENU 3": Value Change {
        n379 = event-data() -> ()  [unwired: 1 in, 6 out]
        n380 = local write "Tab Control"(enum32{"TAB 1", "TAB 2", "TAB 3", "TAB 4"}."TAB 4" ("Tab Control")) -> ()
      }
      event "MENU 4": Value Change {
        n381 = event-data() -> ()  [unwired: 1 in, 6 out]
        n382 = local write "Tab Control"(enum32{"TAB 1", "TAB 2", "TAB 3", "TAB 4"}."TAB 4" ("Tab Control")) -> ()
      }
      event "Back 4": Value Change {
        n383 = event-data() -> ()  [unwired: 1 in, 6 out]
        n384 = local write "Tab Control"(enum32{"TAB 1", "TAB 2", "TAB 3", "TAB 4"}."TAB 1" ("Tab Control")) -> ()
      }
    }
  }
  n385 = while {
    shift-right: [w626] -> _
    shift-left: "" -> [w628]
    stop <- FALSE stop-if-true
    n386 = event shown="[0] \"Text1\": Value Change" {
      selector: _ -> [_ _ _]
      dyn-events: _ -> [_ _ _]
      timeout: _ -> [_ _ _]
      tunnel: w628 -> [_ _ _]
      tunnel: ["ช่วยด้วย ฉันต้องการความช่วยเหลือ !!!" "ฉันต้องการรับประทานอาหาร" "ฉันมีโรคประจำตัว และรู้สึกอาการกำเริบ !!!"] -> w626
      event "Text1": Value Change {
        n387 = event-data() -> ()  [unwired: 1 in, 6 out]
      }
      event "Text2": Value Change {
        n388 = event-data() -> ()  [unwired: 1 in, 6 out]
      }
      event "Text3": Value Change {
        n389 = event-data() -> ()  [unwired: 1 in, 6 out]
      }
    }
    "String" <- w626
  }
  n390 = call-poly "VISA Configure Serial Port"("VISA resource name"="VISA resource name", "baud rate (9600)"=u32 9600) -> ("VISA resource name out"=w7:refnum<visa-resource-name>, "error out"=w5:errorcluster)  [unwired: 12 in]
  n391 = while {
    shift-right: [w640] -> w6
    shift-left: w7 -> [w641]
    shift-right: [w638] -> w4
    shift-left: w5 -> [w639]
    stop <- FALSE stop-if-true
    n392 = Select(t="a", s="LED", f="b") -> (s? t:f=w635:string)
    n393 = VISA Write(VISA resource name=w641, write buffer=w635, error in (no error)=w639) -> (VISA resource name out=w640:refnum<visa-resource-name>, error out=w638:errorcluster)  [unwired: 1 out]
    n394 = Wait (ms)(milliseconds to wait=u32 5) -> ()  [unwired: 1 out]
  }
  n395 = VISA Close(VISA resource name=w6, error in (no error)=w4) -> ()  [unwired: 1 out]
